vi "Dashboard Main.vi"() -> ()   [LabVIEW 2016]
uses:
  <vilib>/Utility/miscctls.llb/LVRowAndColumnTypeDef.ctl
  <vilib>/event_ctls.llb/eventvkey.ctl
  <vilib>/Rock Robotics/Network Tables/NT Read Boolean.vi
  <vilib>/Rock Robotics/WPI/Dashboard/WPI_DashboardLogging Global.vi
panel:
  in  "Camera Settings Right":T1={"Frame Rate"=30, "Compression"=30, "Size"=1, "DB Camera Config"=FALSE} {"Frame Rate" scale=1.0..30.0; "Compression" scale=100.0..-1.0; "Size" items=["640x480", "320x240", "160x120"]}
  in  "Camera Name Right":string(combo)="No Camera Selection"
  out "Camera Info":cluster{"Mbps LED":bool, "Mbps":dbl, "fps":dbl} {"fps" format="%#.1g"; "Mbps" format="%#.1g"}
  in  "Camera Settings":T1={"Frame Rate"=30, "Compression"=30, "Size"=1, "DB Camera Config"=FALSE} {"Frame Rate" scale=1.0..30.0; "Compression" scale=100.0..-1.0; "Size" items=["640x480", "320x240", "160x120"]}
  in  "TCP":refnum<k5>
  in  "Rec Mode":enum32{"Stop", "Record", "Playback"}(radio)
  out "Robot IP":string
  out "Image Message":string="Timeout in Camera Communications"
  in  "Dashboard Tab":T2(tab)
  in  "Wheel Circumference":dbl=14.0
  in  "?":string(combo)
  out "?":string="CHOOSE AN AUTONOMOUS MODE!!!"
  in  "Select Auto":string(combo)="Select Autonomous ..."
  out "NT Connection":bool
  out "JS1 Z":dbl(slide) scale=-1.0..1.0 scale format="%#_2e"
  out "JS1 Graph":cluster{"X":dbl, "Y":dbl}[](graph)
  out "JS1 Buttons":T3
  out "JS2 Z":dbl(slide) scale=-1.0..1.0 scale format="%#_2e"
  out "JS2 Graph":cluster{"X":dbl, "Y":dbl}[](graph)
  out "JS2 Buttons":T3
  out "Mode":T4(ring)=enum."Auto Disabled"
  out "Camera Image Right":T5(plugin-control)
  out "Gear In?":bool
  in  "?":string="CORTECHS ROBOTICS"
  out "Mid":dbl(slide) scale=0.0..320.0
  out "Targets Found?":bool
  out "Low Gear?":bool
  out "PID On?":bool
  out "?":dbl
  out "Time Remaining":u8(slide) scale=0.0..135.0
  in  "Test Slider":dbl(slide) scale=0.0..100.0 scale format="%#_3g"
  in  "On/Off":bool caption="Solenoid"
  in  "Test Name":u16(ring) items=["Select the test to run..."]
  in  "Test Tree":string(tree)
  in  "Motor":cluster{"Value":dbl, "Enable":bool} {"Value" scale=-1.0..1.0 scale format="%#_3g"}
  out "Progress":T6 {"Test Progress" scale=0.0..100.0}
  in  "Rev/Fwd":cluster{"Forward":bool, "Reverse":bool}
  in  "Test Ring":u16(ring) items=["Monochrome", "Color"]
  out "Cmd Status":string
  in  "Execute Command":bool
  in  "Command Params":string[][](table)
  in  "Command Selection":i32(listbox)
  in  "CheckList":i32(listbox)
  out "Tree":string(tree)
  out "Camera Image":T5(plugin-control)
  out "Background":bool
  in  "Camera Name":string(combo)="No Camera Selection"
  # "HW"
  # "HW"
  # "Joysticks"
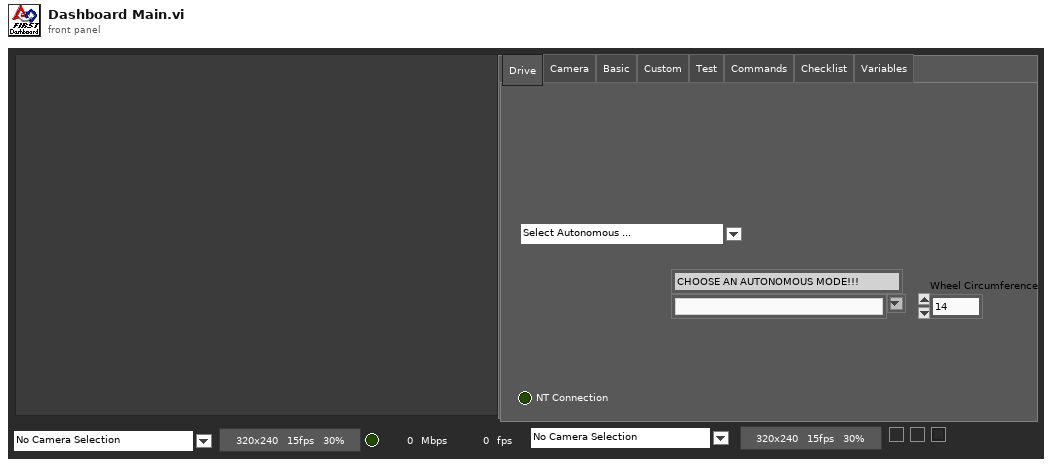
[diagram p1: front panel]
types:
  T1 = cluster{"Frame Rate":i32, "Compression":i32, "Size":u16, "DB Camera Config":bool}
  T2 = enum32{"Drive", "Camera", "Basic", "Custom", "Test", "Commands", "Checklist", "Variables"}
  T3 = cluster{bool, bool, bool, bool, bool, bool, bool, bool, bool, bool, bool, bool}
  T4 = enum8{"Tele-Op Disabled", "Tele-Op Enabled", "Auto Disabled", "Auto Enabled", "Test Disabled", "Test Enabled", "Disconnected", "No Code", "E-Stop"}
  T5 = typedef "IMAQ Image.ctl" = refnum<image>
  T6 = cluster{"Test Progress":u8, "Test Progress Text":string}
  T7 = typedef "Image Type" = u32
  T8 = cluster{"IDs":cluster{"RPC field ID":u16, "Unique ID":u16}, "String":string}
  T9 = enum32{"Drive", "Basic", "Custom", "Test", "Checklist", "Variables"}
  T10 = cluster{"Error Strings":string, "Disable Counts":cluster{u16, u16}, "Rail Faults":cluster{u16, u16, u16}, "Robot IP":string, "DB Mode":u8, "Event Info":cluster{"Name":string, "Type":u8, "Number":u16, "Replay":u8}}
  T11 = cluster{"Storage":cluster{"Disk Free":u64, "RAM Block":u32, "RAM free":u32}, "CPU Utilization":cluster{"CPU % ISR":sgl, "CPU % Time Crit":sgl, "CPU % Timed Str":sgl, "CPU % High":sgl, "CPU % Above":sgl, "CPU % Normal":sgl, "CPU % Low":sgl}, "CAN":cluster{"% Bus Utilization":sgl, "Bus Off Cnt":u32, "TX_FIFO Full Cnt":u32, "Receive Error Cnt":u8, "Transmit Error Cnt":u8}, "HID":cluster{"HID Outputs":u32, "Rumble Low":u16, "Rumble High":u16}[]}
  T12 = cluster{"Status bits":cluster{"Test Mode":bool, "Autonomous":bool, "Enabled":bool, "Code Start":bool, "Brownout":bool, "Reserved 2":bool, "Reserved 3":bool, "E-Stop":bool}, "Code Trace":cluster{"Disabled":bool, "TeleOp":bool, "Auto":bool, "Test":bool}, "Controller Type":enum16{"unknown", "cRIO", "roboRio"}, "Code?":enum16{"unknown", "noCode", "code"}, "Battery V":dbl}
  T13 = cluster{"Control Bits":cluster{"TestMode":bool, "Autonomous":bool, "Enabled":bool, "FMS Present":bool, bool, bool, bool, "E-Stop":bool}, "Team Station ":u8, "Countdown":sgl, "Joystick Values":cluster{"Axes":dbl[], "Buttons":bool[], "POVs":i16[]}[]}
  T14 = cluster{"Axes":dbl[], "Buttons":bool[], "POVs":i16[]}[]
  T15 = cluster{"Axes":dbl[], "Buttons":bool[], "POVs":i16[]}
  T16 = cluster{"Buttons[0]":bool, "Buttons[1]":bool, "Buttons[2]":bool, "Buttons[3]":bool, "Buttons[4]":bool, "Buttons[5]":bool, "Buttons[6]":bool, "Buttons[7]":bool, "Buttons[8]":bool, "Buttons[9]":bool, "Buttons[10]":bool, "Buttons[11]":bool}
  T17 = cluster{"Camera Image":refnum<vi>, "Dashboard Tab":refnum<vi>, "Background":refnum<vi>, "Rec Mode":refnum<vi>, "Test Slider":refnum<vi>, "On/Off ":refnum<vi>, "Test Ring":refnum<vi>, "Rev/Fwd":refnum<vi>, "Test Name":refnum<vi>, "Motor":refnum<vi>, "Progress":refnum<vi>, "CheckList":refnum<vi>, "Tree":refnum<vi>, "Test Tree":refnum<vi>, "Command Params":refnum<vi>, "Command Selection":refnum<vi>, "Execute Command":refnum<vi>, "Cmd Status":refnum<vi>, "Camera Settings":refnum<vi>, "Camera Name":refnum<vi>, "Camera Info":refnum<vi>, "Camera Settings Right":refnum<vi>, "Camera Name Right":refnum<vi>, "Camera Image Right":refnum<vi>}
  T18 = cluster{"Operation":enum16{"Update", "Clear"}, "Color Box":u32}[]
  T19 = typedef "eventvkey.ctl" = enum16{"ASCII", "Enter", "Return", "Shift", "Ctrl", "Alt", "Cmd", "Opt", "Caps", "NumLock", "Clear", "Break", "Up", "Down", "Left", "Right", "Insert", "Delete", "Home", "End", "PageUp", "PageDown", "Escape", "Help", "Pause", "ScrollLock", "F1", "F2", "F3", "F4", "F5", "F6", "F7", "F8", "F9", "F10", "F11", "F12", "F13", "F14", "F15", "F16", "F17", "F18", "F19", "F20", "F21", "F22", "F23", "F24", "Play", "VolumeUp", "VolumeDown", "Mute", "Two Byte Char"}
  T20 = cluster{"Image Size":bool, "Image Type":bool, "Pixel Value":bool, "ROI Information":bool, "Zoom Factor":bool}
  T21 = cluster{"Operation":enum16{"Update", "Clear"}, "Color Box":u32}
  T22 = typedef "LVRowAndColumnTypeDef.ctl" = cluster{"Row":i32, "Column":i32}
  T23 = cluster{"Shift":bool, "Ctrl":bool, "Alt":bool, "Cmd":bool, "Opt":bool}
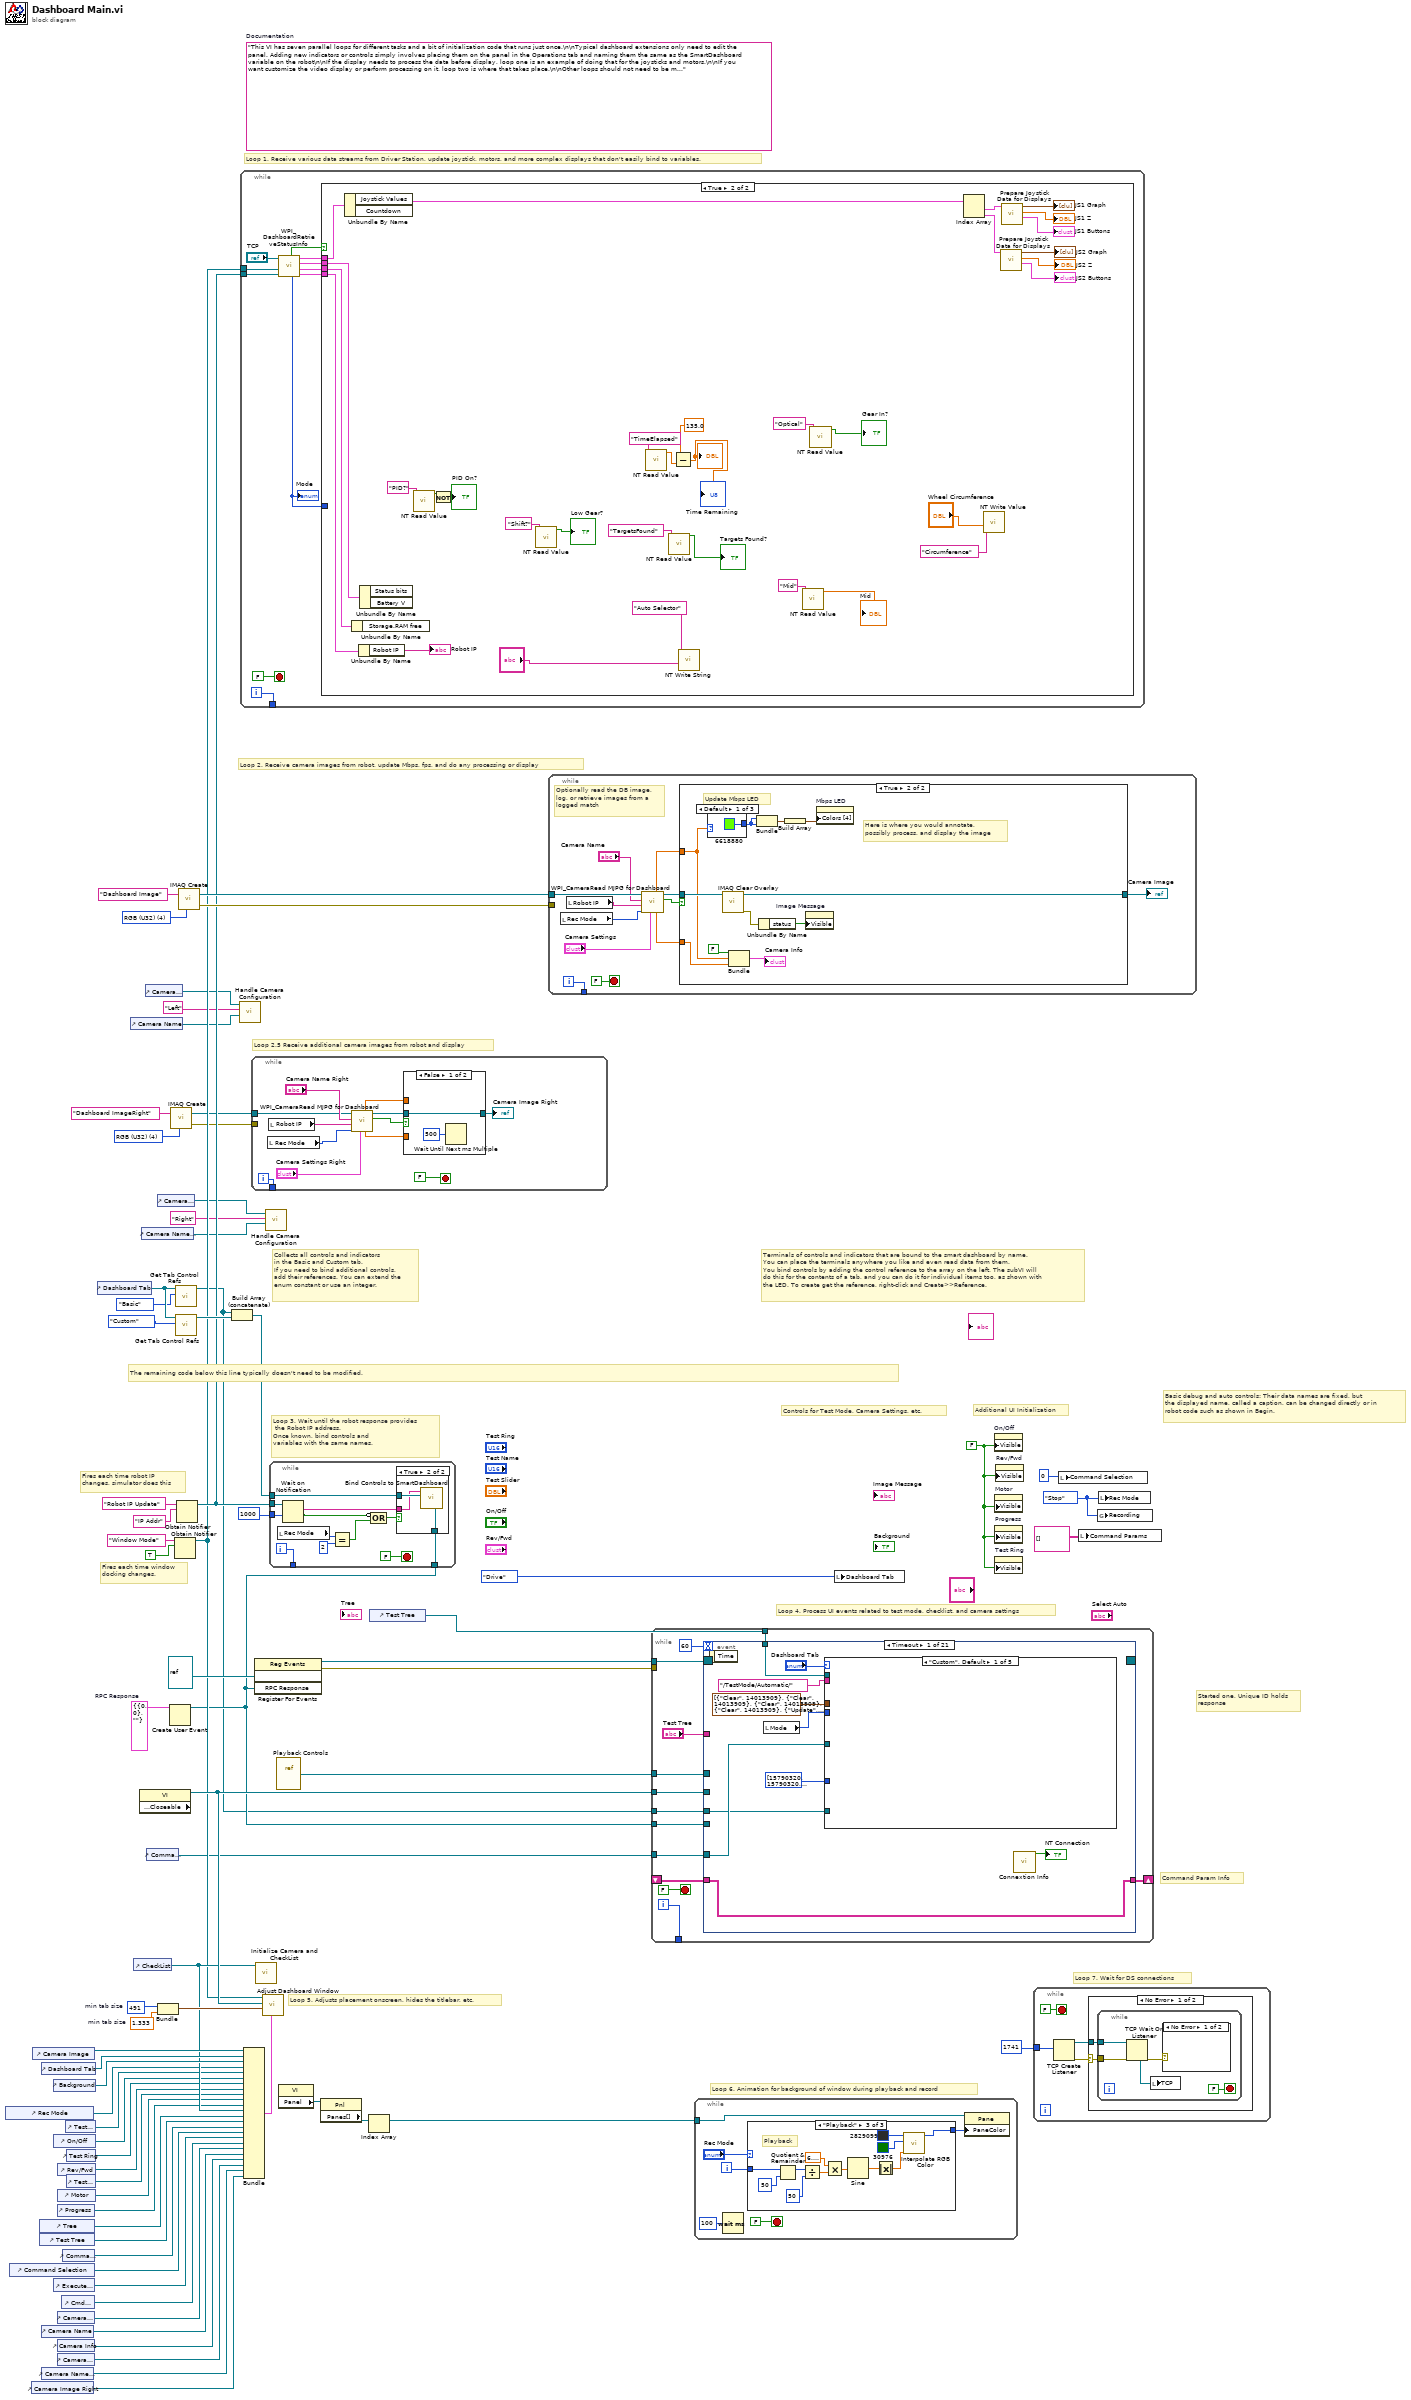
[diagram p0: block diagram]
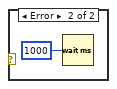
[diagram p3: hidden frame]
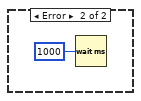
[diagram p4: hidden frame]
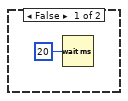
[diagram p5: hidden frame]
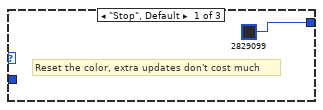
[diagram p6: hidden frame]
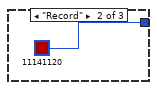
[diagram p7: hidden frame]
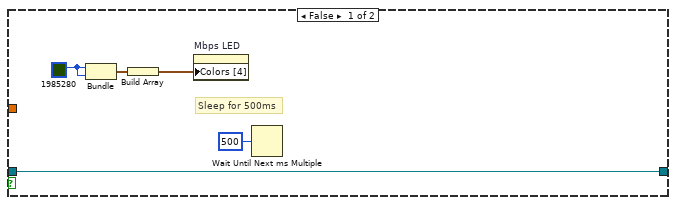
[diagram p9: hidden frame]
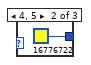
[diagram p10: hidden frame]
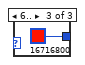
[diagram p11: hidden frame]
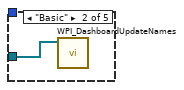
[diagram p12: hidden frame]
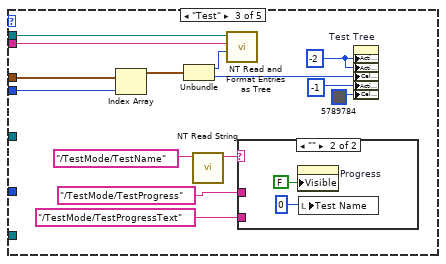
[diagram p13: hidden frame]
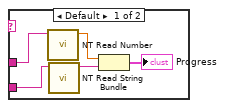
[diagram p14: hidden frame]
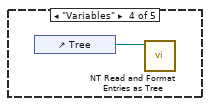
[diagram p15: hidden frame]
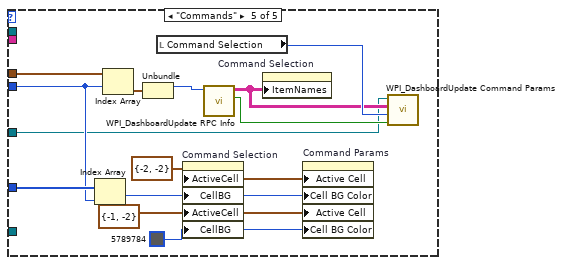
[diagram p16: hidden frame]
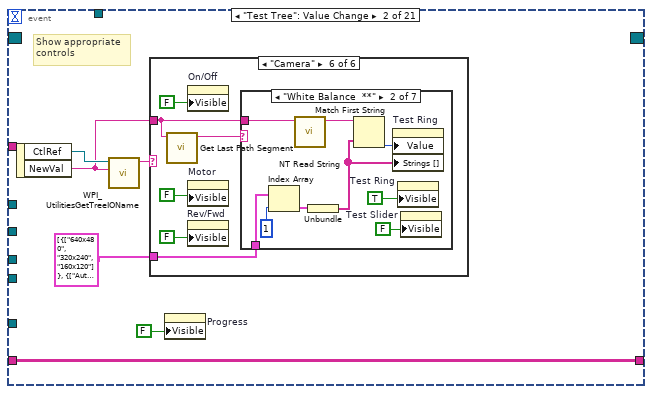
[diagram p17: hidden frame]
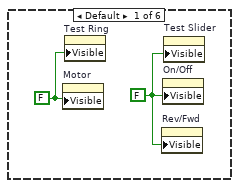
[diagram p18: hidden frame]
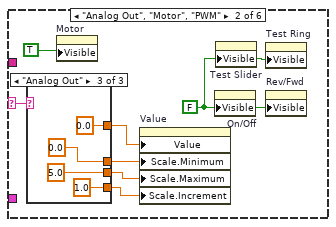
[diagram p19: hidden frame]
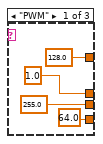
[diagram p20: hidden frame]
diagram:
  w10 = T7 4 items=["Grayscale (U8)", "Grayscale (I16)", "Grayscale (SGL)", "Complex (CSG)", "RGB (U32)", "HSL (U32)", "RGB (U64)"] ("Image Type")
  w24 = T8 {"IDs"={"RPC field ID"=0, "Unique ID"=0}, "String"=""}  # RPC Response
  w49 = 491  # min tab size
  w48 = 1.333  # min tab size
  w56 = enum32{"Stop", "Record", "Playback"}."Stop" ("Rec Mode")
  w31 = FALSE ("Visible")
  (unwired) "This VI has seven parallel loops for different tasks and a bit of initialization code that runs just once.\n\nTypical dashboard extensions only need to edit the panel. Adding new indicators or controls simply involves placing them on the panel in the Operations tab and naming them the same as the SmartDashboard variable on the robot\n\nIf the display needs to process the data before display, loop one is an example of doing that for the joysticks and motors.\n\nIf you want customize the video display or perform processing on it, loop two is where that takes place.\n\nOther loops should not need to be modified. They are pretty standard, and document the task they perform."  # Documentation
  w73 = T7 4 items=["Grayscale (U8)", "Grayscale (I16)", "Grayscale (SGL)", "Complex (CSG)", "RGB (U32)", "HSL (U32)", "RGB (U64)"] ("Image Type")
  # "Loop 2.5 Receive additional camera images from robot and display"
  # "Command Param Info"
  # "Started one, Unique ID holds\nresponse"
  # "Loop 7. Wait for DS connections"
  # "Basic debug and auto controls: Their data names are fixed, but\nthe displayed name, called a caption, can be changed directly or in\nrobot code such as shown in Begin."
  # "Controls for Test Mode, Camera Settings, etc."
  # "Additional UI Initialization"
  # "Loop 6. Animation for background of window during playback and record"
  # "Fires each time robot IP\nchanges, simulator does this"
  # "Fires each time window\ndocking changes."
  # "Collects all controls and indicators\nin the Basic and Custom tab.\nIf you need to bind additional controls,\nadd their references. You can extend the\nenum constant or use an integer."
  # "The remaining code below this line typically doesn't need to be modified."
  # "Loop 4. Process UI events related to test mode, checklist, and camera settings"
  # "Terminals of controls and indicators that are bound to the smart dashboard by name.\nYou can place the terminals anywhere you like and even read data from them.\nYou bind controls by adding the control reference to the array on the left. The subVI will\ndo this for the contents of a tab, and you can do it for individual items too, as shown with\nthe LED. To create get the reference, right-click and Create>>Reference."
  # "Loop 3. Wait until the robot response provides\n the Robot IP address.\nOnce known, bind controls and\nvariables with the same names."
  # "Loop 5. Adjusts placement onscreen, hides the titlebar, etc."
  # "Loop 1. Receive various data streams from Driver Station, update joystick, motors, and more complex displays that don't easily bind to variables."
  # "Loop 2. Receive camera images from robot, update Mbps, fps, and do any processing or display"
  n1 = control-ref of="Rec Mode"() -> (w37:refnum<vi>)
  n2 = control-ref of="Command Selection"() -> (w23:refnum<vi>)
  n3 = control-ref of="Camera Image Right"() -> (w1:refnum<vi>)
  n4 = control-ref of="Camera Image"() -> (w51:refnum<vi>)
  n5 = control-ref of="Tree"() -> (w41:refnum<vi>)
  n6 = control-ref of="Test Tree"() -> (w40:refnum<vi>)
  n7 = control-ref of="Dashboard Tab"() -> (w50:refnum<vi>)
  n8 = control-ref of="Camera Name"() -> (w14:refnum<vi>)
  n9 = control-ref of="Camera Name Right"() -> (w2:refnum<vi>)
  n10 = control-ref of="Execute Command"() -> (w25:refnum<vi>)
  n11 = control-ref of="Background"() -> (w46:refnum<vi>)
  n12 = control-ref of="On/Off"() -> (w35:refnum<vi>)
  n13 = control-ref of="Progress"() -> (w32:refnum<vi>)
  n14 = control-ref of="Camera Settings"() -> (w15:refnum<vi>)
  n15 = control-ref of="Camera Info"() -> (w13:refnum<vi>)
  n16 = control-ref of="Camera Settings Right"() -> (w3:refnum<vi>)
  n17 = control-ref of="Rev/Fwd"() -> (w33:refnum<vi>)
  n18 = control-ref of="Motor"() -> (w38:refnum<vi>)
  n19 = control-ref of="Cmd Status"() -> (w19:refnum<vi>)
  n20 = control-ref of="Command Params"() -> (w26:refnum<vi>)
  n21 = control-ref of="Test Slider"() -> (w36:refnum<vi>)
  n22 = control-ref of="Test Ring"() -> (w34:refnum<vi>)
  n23 = control-ref of="Test Name"() -> (w39:refnum<vi>)
  n24 = control-ref of="Dashboard Tab"() -> (w54:refnum<vi>)
  n25 = control-ref of="Camera Name"() -> (w16:refnum<vi>)
  n26 = control-ref of="CheckList"() -> (w42:refnum<vi>)
  n27 = property class="VI" props=["Front Panel.Closeable"]() -> (reference out=w55:refnum<vi>)  [unwired: 2 in, 2 out]
  n28 = control-ref of="Camera Name Right"() -> (w6:refnum<vi>)
  n29 = control-ref of="Camera Settings"() -> (w17:refnum<vi>)
  n30 = control-ref of="Command Params"() -> (w18:refnum<vi>)
  n31 = control-ref of="Camera Settings Right"() -> (w7:refnum<vi>)
  n32 = Bundle("min tab size"=w49, "min tab size"=w48) -> (w47:cluster{"min tab size":i32, "min tab size":dbl})  [unwired: 1 in]
  n33 = Create User Event(user event datatype=w24) -> (user event=w20:refnum<user-event>)  [unwired: 1 in, 1 out]
  n34 = call "IMAQ Create"("Image Name"="Dashboard ImageRight", "Image Type"=w10) -> ("New Image"=w9:T5, "error out"=w8:errorcluster)  [unwired: 2 in, 1 out]
  n35 = Obtain Notifier(name (unnamed)="Window Mode", notification data type=TRUE) -> (notifier out=w29:refnum<notifier>)  [unwired: 2 in, 2 out]
  n36 = call <vilib>:"Get Tab Control Refs.vi"("Page Index"=T9."Basic" ("Dashboard Tab"), "TabControl in"=w54) -> ("ControlsOnPage"=w12:refnum<vi>[])  [unwired: 9 in]
  n37 = call <vilib>:"Get Tab Control Refs.vi"("Page Index"=T9."Custom" ("Dashboard Tab"), "TabControl in"=w54) -> ("ControlsOnPage"=w53:refnum<vi>[])  [unwired: 9 in]
  n38 = Obtain Notifier(name (unnamed)="Robot IP Update", notification data type="IP Addr" ("name (unnamed)")) -> (notifier out=w30:refnum<notifier>)  [unwired: 2 in, 2 out]
  n39 = call "IMAQ Create"("Image Name"="Dashboard Image", "Image Type"=w73) -> ("New Image"=w71:T5, "error out"=w70:errorcluster)  [unwired: 2 in, 1 out]
  n40 = Build Array (concatenate)(w12, w53) -> (w52:refnum<vi>[])
  n41 = call "Handle Camera Configuration.vi"("CameraNameRef"=w16, "Camera File Name"="Left", "ClusterRef"=w17) -> ()  [unwired: 9 in]
  n42 = while {
    tunnel: [w83] -> _
    tunnel: w30 -> [w77]
    tunnel: w29 -> [w74]
    i -> [w83]
    stop <- FALSE stop-if-true
    n43 = call <vilib>:"WPI_DashboardRetrieveStatusInfo.vi"("Binding Refnum"=w77, "Window Mode Notifier"=w74, "TCP Cnx"="TCP") -> ("Power and Errors"=w78:T10, "Robot Metrics"=w81:T11, "Status Info"=w82:T12, "Control Info"=w79:T13, "Robot Mode"=w76:T4, "Process?"=w80:bool)  [unwired: 3 in]
    "Mode" <- w76
    n44 = case shown="True" w80 {
      tunnel: w82 -> [_ w118]
      tunnel: w81 -> [_ w117]
      tunnel: w79 -> [_ w116]
      tunnel: w78 -> [_ w115]
      tunnel: w76 -> [_ _]
      frame False {
        n45 = Wait (ms)(milliseconds to wait=u32 20) -> ()  [unwired: 1 out]
      }
      frame True {
        n46 = Unbundle By Name(w116) -> ("Joystick Values"=w114:T14)  [unwired: 1 out]
        n47 = Unbundle By Name(w117) -> ()  [unwired: 1 out]
        n48 = Unbundle By Name(w115) -> ("Robot IP"=→"Robot IP":string)
        n49 = Unbundle By Name(w118) -> ()  [unwired: 2 out]
        n50 = call-poly <vilib>:"NT Read Value.vi"("Name"="PID?") -> ("Boolean"=w101:bool)  [unwired: 9 in, 1 out]
        n51 = Not(x=w101) -> (.not. x?=→"PID On?":bool)
        n52 = call-poly <vilib>:"NT Read Value.vi"("Name"="Shift?") -> ("Boolean"=→"Low Gear?":bool)  [unwired: 9 in, 1 out]
        n53 = call-poly <vilib>:"NT Read Value.vi"("Name"="TimeElapsed") -> ("Numeric"=w95:dbl)  [unwired: 9 in, 1 out]
        n54 = call-poly <vilib>:"NT Read Value.vi"("Name"="TargetsFound") -> ("Boolean"=→"Targets Found?":bool)  [unwired: 9 in, 1 out]
        n55 = Subtract(x=135.0, y=w95) -> (x-y=→"Time Remaining" →"?":dbl)
        n56 = call <vilib>:"NT Write String.vi"("String"="?", "Name"="Auto Selector") -> ()  [unwired: 9 in, 1 out]
        n57 = call-poly <vilib>:"NT Read Value.vi"("Name"="Mid") -> ("Numeric"=→"Mid":dbl)  [unwired: 9 in, 1 out]
        n58 = call-poly <vilib>:"NT Read Value.vi"("Name"="Optical") -> ("Boolean"=→"Gear In?":bool)  [unwired: 9 in, 1 out]
        n59 = Index Array(array=w114) -> (element #1=w113:T15, element #2=w109:T15)  [unwired: 2 in]
        n60 = call-poly <vilib>:"NT Write Value.vi"("Numeric"="Wheel Circumference", "Name"="Circumference") -> ()  [unwired: 9 in, 1 out]
        n61 = call "Prepare Joystick Data for Displays.vi"("Joystick Values"=w109) -> ("Buttons"=→"JS2 Buttons":T16, "Z Axis"=→"JS2 Z":dbl, "Cartesian Data"=→"JS2 Graph":cluster{"X axis":dbl, "X axis":dbl}[])  [unwired: 8 in]
        n62 = call "Prepare Joystick Data for Displays.vi"("Joystick Values"=w113) -> ("Buttons"=→"JS1 Buttons":T16, "Z Axis"=→"JS1 Z":dbl, "Cartesian Data"=→"JS1 Graph":cluster{"X axis":dbl, "X axis":dbl}[])  [unwired: 8 in]
      }
    }
  }
  n63 = Bundle("Camera Image"=w51, "Dashboard Tab"=w50, "Background"=w46, "Rec Mode"=w37, "Test Slider"=w36, "On/Off"=w35, "Test Ring"=w34, "Rev/Fwd"=w33, "Test Name"=w39, "Motor"=w38, "Progress"=w32, "CheckList"=w42, "Tree"=w41, "Test Tree"=w40, "Command Params"=w26, "Command Selection"=w23, "Execute Command"=w25, "Cmd Status"=w19, "Camera Settings"=w15, "Camera Name"=w14, "Camera Info"=w13, "Camera Settings Right"=w3, "Camera Name Right"=w2, "Camera Image Right"=w1) -> (w43:T17)  [unwired: 1 in]
  n64 = while {
    tunnel: w9 -> [w129]
    tunnel: w8 -> [_]
    tunnel: [w123] -> _
    i -> [w123]
    stop <- FALSE stop-if-true
    n65 = local read "Rec Mode"() -> (w127:enum32{"Stop", "Record", "Playback"})
    n66 = local read "Robot IP"() -> (w128:string)
    n67 = call <vilib>:"WPI_CameraRead MJPG for Dashboard.vi"("Camera Settings"="Camera Settings Right", "Rec Mode"=w127, "Robot IP"=w128, "Camera Name"="Camera Name Right", "Refnum in"=w129) -> ("Active"=w122:bool, "Refnum out"=w125:T5, "FPS"=w120:dbl, "Bandwidth (Mbps)"=w121:dbl)  [unwired: 3 in]
    n68 = case shown="False" w122 {
      tunnel: w125 -> [w131 w133]
      tunnel: w121 -> [_ _]
      tunnel: w120 -> [_ _]
      tunnel: [w131 w133] -> w119
      frame False {
        n69 = Wait Until Next ms Multiple(millisecond multiple=u32 500) -> ()  [unwired: 1 out]
      }
      frame True {
      }
    }
    "Camera Image Right" <- w119
  }
  n70 = register-events(refnum<vi> refnum, w20) -> (reference out=w60:refnum<event-registration>, error out=w59:errorcluster)  [unwired: 2 in]
  n71 = call "Initialize Camera and CheckList.vi"("ListBox in"=w42) -> ()  [unwired: 11 in]
  n72 = call "Adjust Dashboard Window.vi"("Sizing Refnums"=w43, "Size Constraints"=w47, "VI"=w55, "WIn Mode"=w29) -> ()  [unwired: 8 in]
  n73 = call "Handle Camera Configuration.vi"("CameraNameRef"=w6, "Camera File Name"="Right", "ClusterRef"=w7) -> ()  [unwired: 9 in]
  n74 = while {
    tunnel: w52 -> [w145]
    tunnel: w30 -> [w143]
    tunnel: [w141] -> _
    tunnel: u32 1000 ("milliseconds to wait") -> [w140]
    tunnel: w20 -> [w134]
    i -> [w141]
    stop <- FALSE stop-if-true
    n75 = local read "Rec Mode"() -> (w136:enum32{"Stop", "Record", "Playback"})
    n76 = Wait on Notification(notifier=w143, timeout in ms (-1)=w140) -> (notification=w142:string, timed out?=w138:bool)  [unwired: 2 in, 2 out]
    n77 = Equal?(x=w136, y=u16 2 ("Rec Mode")) -> (x = y?=w137:bool)
    n78 = Compound Arithmetic op=OR(invert w138, w137) -> (w139:bool)
    n79 = case shown="True" w139 {
      tunnel: w145 -> [_ w148]
      tunnel: w142 -> [_ w147]
      tunnel: w134 -> [_ w146]
      frame False {
      }
      frame True {
        n80 = call <vilib>:"Bind Controls to SmartDashboard.vi"("RPC ref"=w146, "Bound Control Refs"=w148, "Server IP Address"=w147) -> ()  [unwired: 9 in]
      }
    }
  }
  n81 = vi-ref "Playback Controls.vi"() -> (w61:refnum<vi>)
  n82 = property class="VI"() -> ("Panel"=w63:refnum<vi>)  [unwired: 2 in, 2 out]
  n83 = property class="Pnl"(reference=w63) -> ("Panes[]"=w64:refnum<vi>[])  [unwired: 1 in, 2 out]
  n84 = Index Array(array=w64) -> (element=w62:refnum<vi>)  [unwired: 1 in]
  n85 = control-ref of="Test Tree"() -> (w65:refnum<vi>)
  n86 = while {
    tunnel: w71 -> [w158]
    tunnel: w70 -> [_]
    tunnel: [w159] -> _
    i -> [w159]
    stop <- FALSE stop-if-true
    # "Optionally read the DB image,\nlog, or retrieve images from a\nlogged match"
    n87 = local read "Rec Mode"() -> (w154:enum32{"Stop", "Record", "Playback"})
    n88 = local read "Robot IP"() -> (w153:string)
    n89 = call <vilib>:"WPI_CameraRead MJPG for Dashboard.vi"("Camera Settings"="Camera Settings", "Rec Mode"=w154, "Robot IP"=w153, "Camera Name"="Camera Name", "Refnum in"=w158) -> ("Active"=w156:bool, "Refnum out"=w157:T5, "FPS"=w155:dbl, "Bandwidth (Mbps)"=w152:dbl)  [unwired: 3 in]
    n90 = case shown="True" w156 {
      tunnel: w157 -> [w161 w172]
      tunnel: w152 -> [_ w169]
      tunnel: w155 -> [_ w170]
      tunnel: [w161 w166] -> w149
      frame False {
        w163 = u32 1985280 ("Color Box")
        # "Sleep for 500ms"
        n91 = Bundle("Color Box"=w163, "Color Box"=w163) -> (w164:cluster{"Color Box":u32, "Color Box":u32})  [unwired: 1 out]
        n92 = Build Array(w164) -> (w162:cluster{"Color Box":u32, "Color Box":u32}[])
        n93 = property on="Mbps LED" class="Bool (strict)"("Colors [4]"=w162) -> ()  [unwired: 2 in, 2 out]
        n94 = Wait Until Next ms Multiple(millisecond multiple=u32 500) -> ()  [unwired: 1 out]
      }
      frame True {
        # "Here is where you would annotate,\npossibly process, and display the image"
        # "Update Mbps LED"
        n95 = case shown="Default" w169 {
          tunnel: [u32 6618880 ("Color Box") u32 16776722 ("Color Box") u32 16716800 ("Color Box")] -> w173
          frame Default {
          }
          frame 4, 5 {
          }
          frame 6.. {
          }
        }
        n96 = call "IMAQ Clear Overlay"("Image"=w172) -> ("error out"=w175:errorcluster, "Image Out"=w166:T5)  [unwired: 2 in, 7 out]
        n97 = Bundle(FALSE, "Bandwidth (Mbps)"=w169, "FPS"=w170) -> (→"Camera Info":cluster{bool, "Bandwidth (Mbps)":dbl, "FPS":dbl})  [unwired: 1 in]
        n98 = Bundle("Color Box"=w173, "Color Box"=w173) -> (w174:cluster{"Color Box":u32, "Color Box":u32})  [unwired: 1 out]
        n99 = Unbundle By Name(w175) -> ("status"=w176:bool)
        n100 = Build Array(w174) -> (w171:cluster{"Color Box":u32, "Color Box":u32}[])
        n101 = property on="Image Message" class="Str"("Visible"=w176) -> ()  [unwired: 2 in, 2 out]
        n102 = property on="Mbps LED" class="Bool (strict)"("Colors [4]"=w171) -> ()  [unwired: 2 in, 2 out]
      }
    }
    "Camera Image" <- w149
  }
  n103 = while {
    tunnel: [w189] -> _
    tunnel: w65 -> [w188]
    tunnel: w61 -> [w187]
    tunnel: w60 -> [w186]
    tunnel: w59 -> [_]
    tunnel: w55 -> [w185]
    tunnel: w20 -> [w184]
    tunnel: w18 -> [w183]
    shift-right: [w182] -> _
    shift-left: _ -> [w181]
    tunnel: w12 -> [w180]
    i -> [w189]
    stop <- FALSE stop-if-true
    n104 = event shown="[0] Timeout" {
      selector: w186 -> [_ _ _ _ _ _ _ _ _ _ _ _ _ _ _ _ _ _ _ _ _]
      dyn-events: [_ _ _ _ _ _ _ _ _ _ _ _ _ _ _ _ w445 _ _ _ _] -> _
      timeout: u32 60 ("milliseconds to wait") -> [_ _ _ _ _ _ _ _ _ _ _ _ _ _ _ _ _ _ _ _ _]
      tunnel: w188 -> [w201 _ _ _ _ _ _ _ _ _ _ _ _ _ _ _ _ _ _ _ _]
      tunnel: "Test Tree" -> [_ _ _ _ _ _ _ _ _ _ _ w412 w420 w422 w426 w434 _ _ _ _ _]
      tunnel: w187 -> [_ _ _ _ _ _ _ _ _ _ _ _ _ _ _ _ w447 _ w465 _ _]
      tunnel: w185 -> [_ _ _ _ _ _ _ _ _ _ _ _ _ _ _ _ w443 _ _ _ _]
      tunnel: w184 -> [_ _ _ _ _ _ _ _ _ _ _ _ _ _ _ _ w439 _ _ _ _]
      tunnel: w183 -> [w196 _ _ _ _ _ w363 _ _ _ _ _ _ _ _ _ _ _ _ _ _]
      tunnel: [w195 w240 w342 w347 w356 w360 w361 w370 w380 w387 w399 w411 w418 w421 w425 w433 w438 w460 w462 w466 w477] -> w182
      tunnel: w181 -> [w195 w240 w342 w347 w356 w360 w361 _ _ w387 w399 w411 w418 w421 w425 w433 w438 w460 w462 w466 w477]
      tunnel: w180 -> [w193 _ _ _ _ _ _ _ _ _ _ _ _ _ _ _ _ _ _ _ _]
      event Timeout {
        n105 = event-data() -> ()  [unwired: 1 in, 1 out]
        n106 = local read "Mode"() -> (w198:T4)
        n107 = case shown="\"Custom\", Default" "Dashboard Tab" {
          tunnel: w201 -> [_ _ w217 _ _]
          tunnel: "/TestMode/Automatic/" ("Name Pattern") -> [_ _ w216 _ _]
          tunnel: T18 [{"Operation"=enum."Clear", "Color Box"=14013909}, {"Operation"=enum."Clear", "Color Box"=14013909}, {"Operation"=enum."Clear", "Color Box"=14013909}, {"Operation"=enum."Clear", "Color Box"=14013909}, {"Operation"=enum."Update", "Color Box"=14013909}, {"Operation"=enum."Update", "Color Box"=16777215}, {"Operation"=enum."Clear", "Color Box"=14013909}, {"Operation"=enum."Clear", "Color Box"=14013909}, {"Operation"=enum."Clear", "Color Box"=14013909}] -> [_ _ w209 _ w233]
          tunnel: w198 -> [_ _ w208 _ w232]
          tunnel: u32[] [15790320, 15790320, 15790320, 15790320, 16777215, 16777215, 15790320, 15790320, 15790320] -> [_ _ _ _ w238]
          tunnel: w196 -> [_ _ _ _ w226]
          tunnel: w193 -> [_ w203 _ _ _]
          frame "Custom", Default {
          }
          frame "Basic" {
            n108 = call <vilib>:"WPI_DashboardUpdateNames.vi"("Controls on Tab"=w203) -> ()  [unwired: 11 in]
          }
          frame "Test" {
            w215 = -2 ("Active Item:Row Number")
            n109 = Index Array(array=w209, index=w208) -> (element=w210:T21)
            n110 = Unbundle(w210) -> ("Operation"=w211:enum16{"Update", "Clear"}, "Color Box"=w212:u32)
            n111 = call <vilib>:"NT Read String.vi"("Name"="/TestMode/TestName") -> ("String"=w206:string)  [unwired: 9 in, 1 out]
            n112 = call <vilib>:"NT Read and Format Entries as Tree.vi"("Operation"=w211, "Name Pattern"=w216, "Tree Refnum"=w217) -> ()  [unwired: 7 in, 2 out]
            n113 = case shown="\"\"" w206 {
              tunnel: "/TestMode/TestProgress" ("Name") -> [w219 _]
              tunnel: "/TestMode/TestProgressText" ("Name") -> [w218 _]
              frame Default {
                n114 = call <vilib>:"NT Read Number.vi"("Name"=w219) -> ("Numeric"=w220:dbl)  [unwired: 9 in, 1 out]
                n115 = call <vilib>:"NT Read String.vi"("Name"=w218) -> ("String"=w221:string)  [unwired: 9 in, 1 out]
                n116 = Bundle("Numeric"=w220, "String"=w221) -> (→"Progress":cluster{"Numeric":dbl, "String":string})  [unwired: 1 in]
              }
              frame "" {
                n117 = property on="Progress" class="Clust (strict)"("Visible"=FALSE) -> ()  [unwired: 2 in, 2 out]
                n118 = local write "Test Name"(u16 0) -> ()
              }
            }
            n119 = property on="Test Tree" class="Tree (strict)"("Active Item Row Number"=w215, "ActiveColNum"=w215, "CellBG"=w212, "Active Item Row Number"=-1 ("Active Item:Row Number"), "CellBG"=u32 5789784 ("Color Box")) -> ()  [unwired: 2 in, 2 out]
          }
          frame "Variables" {
            n120 = control-ref of="Tree"() -> (w225:refnum<vi>)
            n121 = call <vilib>:"NT Read and Format Entries as Tree.vi"("Tree Refnum"=w225) -> ()  [unwired: 9 in, 2 out]
          }
          frame "Commands" {
            w234 = u32 5789784 ("Color Box")
            w235 = T22 {"Row"=-1, "Column"=-2} ("Active Cell:Active Cell")
            w237 = T22 {"Row"=-2, "Column"=-2} ("Active Cell:Active Cell")
            n122 = Index Array(array=w238, index=w232) -> (element=w236:u32)
            n123 = Index Array(array=w233, index=w232) -> (element=w231:T21)
            n124 = Unbundle(w231) -> ("Operation"=w230:enum16{"Update", "Clear"})  [unwired: 1 out]
            n125 = local read "Command Selection"() -> (w229:i32)
            n126 = property on="Command Selection" class="MCListbox (strict)"("ActiveCell"=w237, "CellBG"=w236, "ActiveCell"=w235, "CellBG"=w234) -> ()  [unwired: 2 in, 2 out]
            n127 = call <vilib>:"WPI_DashboardUpdate RPC Info.vi"("Operation"=w230) -> ("update"=w228:bool, "commands"=w227:string[][])  [unwired: 9 in]
            n128 = property on="Command Selection" class="MCListbox (strict)"("ItemNames"=w227) -> ()  [unwired: 2 in, 2 out]
            n129 = property on="Command Params" class="Tbl (strict)"("Active Cell"=w237, "Cell BG Color"=w236, "Active Cell"=w235, "Cell BG Color"=w234) -> ()  [unwired: 2 in, 2 out]
            n130 = call <vilib>:"WPI_DashboardUpdate Command Params.vi"("Update"=w228, "NewVal"=w229, "Commands"=w227, "Param Tbl"=w226) -> ()  [unwired: 7 in, 1 out]
          }
        }
        n131 = call <vilib>:"Connextion Info.vi"() -> ("Connected"=→"NT Connection":bool)  [unwired: 10 in, 1 out]
      }
      event "Test Tree": Value Change {
        # "Show appropriate\ncontrols"
        n132 = event-data() -> ("CtlRef"=w243:refnum<vi>, "NewVal"=w241:string)  [unwired: 1 in]
        n133 = call <vilib>:"WPI_UtilitiesGetTreeIOName.vi"("NewVal"=w241, "TreeControl in"=w243) -> ("I/O Name"=w244:string)  [unwired: 9 in]
        n134 = case shown="\"Camera\"" w244 {
          selector: w244 -> [_ w251 _ w273 w282 _]
          tunnel: w241 -> [_ _ w270 w272 _ w289]
          tunnel: cluster{string[]}[] [{["640x480", "320x240", "160x120"]}, {["Auto", "Fixed indoor", "Fixed outdoor 1", "Fixed outdoor 2", "Fixed fluorescent 1", "Fixed fluorescent 2", "Hold current"]}, {["Auto", "Flicker-free 50 Hz", "Flicker-free 60 Hz", "Hold current"]}, {["None", "Prioritize frame rate", "Prioritize image quality"]}, {["Monochrome", "Color"]}] -> [_ _ _ _ _ w288]
          frame Default {
            w246 = FALSE ("Visible")
            w245 = FALSE ("Visible")
            n135 = property on="Motor" class="Clust (strict)"("Visible"=w245) -> ()  [unwired: 2 in, 2 out]
            n136 = property on="Test Ring" class="Ring (strict)"("Visible"=w245) -> ()  [unwired: 2 in, 2 out]
            n137 = property on="Rev/Fwd" class="Clust (strict)"("Visible"=w246) -> ()  [unwired: 2 in, 2 out]
            n138 = property on="On/Off" class="Bool (strict)"("Visible"=w246) -> ()  [unwired: 2 in, 2 out]
            n139 = property on="Test Slider" class="Slide (strict)"("Visible"=w246) -> ()  [unwired: 2 in, 2 out]
          }
          frame "Analog Out", "Motor", "PWM" {
            w252 = FALSE ("Visible")
            n140 = case shown="\"Analog Out\"" w251 {
              tunnel: [1.0 ("Value") -1.0 ("Value") 0.0 ("Value")] -> w250
              tunnel: [255.0 ("Value") 1.0 ("Value") 5.0 ("Value")] -> w249
              tunnel: [128.0 ("Value") 0.0 ("Value") 0.0 ("Value")] -> w248
              tunnel: [64.0 ("Value") 0.5 ("Value") 1.0 ("Value")] -> w247
              frame "PWM" {
              }
              frame "Motor", Default {
              }
              frame "Analog Out" {
              }
            }
            n141 = property on="Motor" class="Clust (strict)"("Visible"=TRUE) -> ()  [unwired: 2 in, 2 out]
            n142 = property on="Value" class="Slide (strict)"("Value"=w248, "Scale.Minimum"=w250, "Scale.Maximum"=w249, "Scale.Increment"=w247) -> ()  [unwired: 2 in, 2 out]
            n143 = property on="On/Off" class="Bool (strict)"("Visible"=w252) -> ()  [unwired: 2 in, 2 out]
            n144 = property on="Test Slider" class="Slide (strict)"("Visible"=w252) -> ()  [unwired: 2 in, 2 out]
            n145 = property on="Test Ring" class="Ring (strict)"("Visible"=w252) -> ()  [unwired: 2 in, 2 out]
            n146 = property on="Rev/Fwd" class="Clust (strict)"("Visible"=w252) -> ()  [unwired: 2 in, 2 out]
          }
          frame "Servo" {
            w268 = FALSE ("Visible")
            n147 = call <vilib>:"NT Read Number.vi"("Name"=w270) -> ("Numeric"=w269:dbl)  [unwired: 9 in, 1 out]
            n148 = property on="Test Slider" class="Slide (strict)"("Visible"=TRUE, "Scale.Maximum"=170.0 ("Scale.Range:Maximum")) -> ()  [unwired: 2 in, 2 out]
            n149 = local write "Test Slider"(w269) -> ()
            n150 = property on="Motor" class="Clust (strict)"("Visible"=w268) -> ()  [unwired: 2 in, 2 out]
            n151 = property on="Rev/Fwd" class="Clust (strict)"("Visible"=w268) -> ()  [unwired: 2 in, 2 out]
            n152 = property on="On/Off" class="Bool (strict)"("Visible"=w268) -> ()  [unwired: 2 in, 2 out]
            n153 = property on="Test Ring" class="Ring (strict)"("Visible"=w268) -> ()  [unwired: 2 in, 2 out]
          }
          frame "Relay", "Solenoid" {
            w271 = FALSE ("Visible")
            n154 = property on="Motor" class="Clust (strict)"("Visible"=w271) -> ()  [unwired: 2 in, 2 out]
            n155 = property on="Test Slider" class="Slide (strict)"("Visible"=w271) -> ()  [unwired: 2 in, 2 out]
            n156 = Search and Replace String(input string=w272, search string="/Value  **", replace string="/Direction") -> (result string=w278:string)  [unwired: 5 in, 3 out]
            n157 = property on="Test Ring" class="Ring (strict)"("Visible"=w271) -> ()  [unwired: 2 in, 2 out]
            n158 = call <vilib>:"NT Read String.vi"("Name"=w278) -> ("String"=w276:string)  [unwired: 9 in, 1 out]
            n159 = Equal?(x="Both directions", y=w276) -> (x = y?=w274:bool)
            n160 = Not(x=w274) -> (.not. x?=w275:bool)
            n161 = property on="Rev/Fwd" class="Clust (strict)"("Visible"=w274) -> ()  [unwired: 2 in, 2 out]
            n162 = property on="On/Off" class="Bool (strict)"("Visible"=w275, "Caption.Text"=w273) -> ()  [unwired: 2 in, 2 out]
          }
          frame "Compressor", "Digital Out" {
            w281 = FALSE ("Visible")
            # "Get direction and finish"
            n163 = property on="Motor" class="Clust (strict)"("Visible"=w281) -> ()  [unwired: 2 in, 2 out]
            n164 = property on="Test Slider" class="Slide (strict)"("Visible"=w281) -> ()  [unwired: 2 in, 2 out]
            n165 = property on="Test Ring" class="Ring (strict)"("Visible"=w281) -> ()  [unwired: 2 in, 2 out]
            n166 = property on="On/Off" class="Bool (strict)"("Visible"=TRUE, "Caption.Text"=w282) -> ()  [unwired: 2 in, 2 out]
            n167 = property on="Rev/Fwd" class="Clust (strict)"("Visible"=FALSE) -> ()  [unwired: 2 in, 2 out]
          }
          frame "Camera" {
            n168 = call <vilib>:"Get Last Path Segment.vi"("String in"=w289) -> ("String out"=w290:string)  [unwired: 10 in]
            n169 = property on="On/Off" class="Bool (strict)"("Visible"=FALSE) -> ()  [unwired: 2 in, 2 out]
            n170 = property on="Motor" class="Clust (strict)"("Visible"=FALSE) -> ()  [unwired: 2 in, 2 out]
            n171 = property on="Rev/Fwd" class="Clust (strict)"("Visible"=FALSE) -> ()  [unwired: 2 in, 2 out]
            n172 = case shown="\"White Balance  **\"" w290 {
              tunnel: w289 -> [w296 w305 w314 w323 w332 _ w338]
              tunnel: w288 -> [w294 w302 w311 w320 w329 _ _]
              frame "Size  **" {
                n173 = Index Array(array=w294) -> (element=w293:cluster{string[]})  [unwired: 1 in]
                n174 = call <vilib>:"NT Read String.vi"("Name"=w296) -> ("String"=w295:string)  [unwired: 9 in, 1 out]
                n175 = Unbundle(w293) -> (w291:string[])
                n176 = Match First String(2:w291, 3:w295) -> (0:w292:i32)  [unwired: 1 out]
                n177 = property on="Test Ring" class="Ring (strict)"("Value"=w292, "Strings []"=w291) -> ()  [unwired: 2 in, 2 out]
                n178 = property on="Test Ring" class="Ring (strict)"("Visible"=TRUE) -> ()  [unwired: 2 in, 2 out]
                n179 = property on="Test Slider" class="Slide (strict)"("Visible"=FALSE) -> ()  [unwired: 2 in, 2 out]
              }
              frame "White Balance  **" {
                n180 = Index Array(array=w302, index=1) -> (element=w303:cluster{string[]})
                n181 = call <vilib>:"NT Read String.vi"("Name"=w305) -> ("String"=w304:string)  [unwired: 9 in, 1 out]
                n182 = Unbundle(w303) -> (w300:string[])
                n183 = Match First String(2:w300, 3:w304) -> (0:w299:i32)  [unwired: 1 out]
                n184 = property on="Test Ring" class="Ring (strict)"("Value"=w299, "Strings []"=w300) -> ()  [unwired: 2 in, 2 out]
                n185 = property on="Test Ring" class="Ring (strict)"("Visible"=TRUE) -> ()  [unwired: 2 in, 2 out]
                n186 = property on="Test Slider" class="Slide (strict)"("Visible"=FALSE) -> ()  [unwired: 2 in, 2 out]
              }
              frame "Exposure  **" {
                n187 = Index Array(array=w311, index=2) -> (element=w312:cluster{string[]})
                n188 = call <vilib>:"NT Read String.vi"("Name"=w314) -> ("String"=w313:string)  [unwired: 9 in, 1 out]
                n189 = Unbundle(w312) -> (w308:string[])
                n190 = Match First String(2:w308, 3:w313) -> (0:w309:i32)  [unwired: 1 out]
                n191 = property on="Test Ring" class="Ring (strict)"("Value"=w309, "Strings []"=w308) -> ()  [unwired: 2 in, 2 out]
                n192 = property on="Test Ring" class="Ring (strict)"("Visible"=TRUE) -> ()  [unwired: 2 in, 2 out]
                n193 = property on="Test Slider" class="Slide (strict)"("Visible"=FALSE) -> ()  [unwired: 2 in, 2 out]
              }
              frame "Exposure Priority  **" {
                n194 = Index Array(array=w320, index=3) -> (element=w321:cluster{string[]})
                n195 = call <vilib>:"NT Read String.vi"("Name"=w323) -> ("String"=w322:string)  [unwired: 9 in, 1 out]
                n196 = Unbundle(w321) -> (w317:string[])
                n197 = Match First String(2:w317, 3:w322) -> (0:w318:i32)  [unwired: 1 out]
                n198 = property on="Test Ring" class="Ring (strict)"("Value"=w318, "Strings []"=w317) -> ()  [unwired: 2 in, 2 out]
                n199 = property on="Test Ring" class="Ring (strict)"("Visible"=TRUE) -> ()  [unwired: 2 in, 2 out]
                n200 = property on="Test Slider" class="Slide (strict)"("Visible"=FALSE) -> ()  [unwired: 2 in, 2 out]
              }
              frame "Color Enable  **" {
                n201 = Index Array(array=w329, index=4) -> (element=w330:cluster{string[]})
                n202 = call <vilib>:"NT Read String.vi"("Name"=w332) -> ("String"=w331:string)  [unwired: 9 in, 1 out]
                n203 = Unbundle(w330) -> (w326:string[])
                n204 = Match First String(2:w326, 3:w331) -> (0:w327:i32)  [unwired: 1 out]
                n205 = property on="Test Ring" class="Ring (strict)"("Value"=w327, "Strings []"=w326) -> ()  [unwired: 2 in, 2 out]
                n206 = property on="Test Ring" class="Ring (strict)"("Visible"=TRUE) -> ()  [unwired: 2 in, 2 out]
                n207 = property on="Test Slider" class="Slide (strict)"("Visible"=FALSE) -> ()  [unwired: 2 in, 2 out]
              }
              frame Default {
                n208 = property on="Test Ring" class="Ring (strict)"("Visible"=FALSE) -> ()  [unwired: 2 in, 2 out]
                n209 = property on="Test Slider" class="Slide (strict)"("Visible"=FALSE) -> ()  [unwired: 2 in, 2 out]
              }
              frame "Brightness  **", "Color Level  **", "Compression  **", "FPS  **", "Sharpness  **" {
                n210 = call <vilib>:"NT Read Number.vi"("Name"=w338) -> ("Numeric"=w337:dbl)  [unwired: 9 in, 1 out]
                n211 = local write "Test Slider"(w337) -> ()
                n212 = property on="Test Slider" class="Slide (strict)"("Visible"=TRUE, "Scale.Maximum"=100.0 ("Scale.Range:Maximum")) -> ()  [unwired: 2 in, 2 out]
                n213 = property on="Test Ring" class="Ring (strict)"("Visible"=FALSE) -> ()  [unwired: 2 in, 2 out]
              }
            }
          }
        }
        n214 = property on="Progress" class="Clust (strict)"("Visible"=FALSE) -> ()  [unwired: 2 in, 2 out]
      }
      event "Test Name": Mouse Enter {
        # "Populate the ring with the list of tests"
        n215 = event-data() -> ()  [unwired: 1 in, 1 out]
        n216 = call <vilib>:"NT Read String Array.vi"("Name"="/TestMode/TestList") -> ("String Array"=w346:string[])  [unwired: 9 in, 1 out]
        n217 = Build Array (concatenate)("Select the test to run...", w346) -> (w345:string[])
        n218 = property on="Test Name" class="Ring (strict)"("Strings []"=w345) -> ()  [unwired: 2 in, 2 out]
      }
      event "Test Name": Value Change {
        w348 = FALSE ("Visible")
        # "Tell the robot the test name to run"
        n219 = event-data() -> ("NewVal"=w352:u16)  [unwired: 1 in]
        n220 = property on="Test Name" class="Ring (strict)"() -> ("Strings []"=w353:string[])  [unwired: 2 in, 2 out]
        n221 = local write "Progress"(T6 {"Test Progress"=0, "Test Progress Text"=""} ("Progress")) -> ()
        n222 = Index Array(array=w353, index=w352) -> (element=w351:string)
        n223 = call <vilib>:"NT Write String.vi"("String"=w351, "Name"="/TestMode/TestName") -> ()  [unwired: 9 in, 1 out]
        n224 = property on="Progress" class="Clust (strict)"("Visible"=TRUE) -> ()  [unwired: 2 in, 2 out]
        n225 = property on="Motor" class="Clust (strict)"("Visible"=w348) -> ()  [unwired: 2 in, 2 out]
        n226 = property on="Test Slider" class="Slide (strict)"("Visible"=w348) -> ()  [unwired: 2 in, 2 out]
        n227 = property on="On/Off" class="Bool (strict)"("Visible"=w348) -> ()  [unwired: 2 in, 2 out]
        n228 = property on="Rev/Fwd" class="Clust (strict)"("Visible"=w348) -> ()  [unwired: 2 in, 2 out]
        n229 = property on="Test Ring" class="Ring (strict)"("Visible"=w348) -> ()  [unwired: 2 in, 2 out]
      }
      event "Select Auto": Mouse Enter {
        # "Populate the combo box with the list of autonomous options"
        n230 = event-data() -> ()  [unwired: 1 in, 1 out]
        n231 = call <vilib>:"NT Read String Array.vi"("Name"="Auto List") -> ("String Array"=w355:string[])  [unwired: 9 in, 1 out]
        n232 = property on="Select Auto" class="CmbBox"("Strings[]"=w355) -> ()  [unwired: 2 in, 2 out]
      }
      event "Select Auto": Value Change {
        # "User modified the Auto Selection. Write to NT variable so robot knows."
        n233 = event-data() -> ("NewVal"=w358:string)  [unwired: 1 in]
        n234 = call <vilib>:"NT Write String.vi"("String"=w358, "Name"="Auto Selector") -> ()  [unwired: 9 in, 1 out]
      }
      event "Command Selection": Value Change {
        # "Get the params and show in table"
        n235 = event-data() -> ("NewVal"=w364:i32)  [unwired: 1 in]
        n236 = property on="Command Selection" class="MCListbox (strict)"() -> ("ItemNames"=w362:string[][])  [unwired: 2 in, 2 out]
        n237 = call <vilib>:"WPI_DashboardUpdate Command Params.vi"("NewVal"=w364, "Commands"=w362, "Param Tbl"=w363) -> ()  [unwired: 8 in, 1 out]
      }
      event "Execute Command": Value Change {
        # "Started one, Unique ID holds\nresponse"
        n238 = event-data() -> ()  [unwired: 1 in, 1 out]
        n239 = property on="Command Selection" class="MCListbox (strict)"() -> ("ItemNames"=w375:string[][])  [unwired: 2 in, 2 out]
        n240 = Index Array(array=w375, index (row)="Command Selection", index (col)=0) -> (element=w373:string)
        n241 = call <vilib>:"Invoke Commands.vi"("Command Params"="Command Params", "Function Name"=w373) -> ("Params"=w369:u8, "Started"=w368:bool)  [unwired: 7 in, 1 out]
        n242 = Array Subset(array="Command Params", length (row)=w369) -> (w370:string[][])  [unwired: 3 in]
        n243 = Select(t="Executing" ("Cmd Status"), s=w368, f="" ("Cmd Status")) -> (s? t:f=→"Cmd Status":string)
      }
      event "Command Selection": Double Click {
        n244 = event-data() -> ("Row"=w383:i32)  [unwired: 1 in]
        n245 = property on="Command Selection" class="MCListbox (strict)"() -> ("ItemNames"=w386:string[][])  [unwired: 2 in, 2 out]
        n246 = local read "Command Params"() -> (w382:string[][])
        n247 = Index Array(array=w386, index (row)=w383, index (col)=0) -> (element=w384:string)
        n248 = call <vilib>:"Invoke Commands.vi"("Command Params"=w382, "Function Name"=w384) -> ("Params"=w381:u8, "Started"=w376:bool)  [unwired: 7 in, 1 out]
        n249 = Array Subset(array=w382, length (row)=w381) -> (w380:string[][])  [unwired: 3 in]
        n250 = Select(t="Executing" ("Cmd Status"), s=w376, f="" ("Cmd Status")) -> (s? t:f=w377:string)
        n251 = local write "Cmd Status"(w377) -> ()
      }
      event "CheckList": Double Click {
        # "Shift clears all"
        # "Update symbols on the listbox"
        n252 = event-data() -> ("PlatMods.Shift"=w388:bool, "Row"=w390:i32)  [unwired: 1 in]
        n253 = case shown="True" w388 {
          tunnel: w390 -> [w394 _]
          tunnel: 1 -> [w393 _]
          frame False {
            n254 = property on="CheckList" class="LstBox (strict)"() -> ("Item Symbols"=w392:i32[])  [unwired: 2 in, 2 out]
            n255 = Replace Array Subset(array=w392, new element=w393, index=w394) -> (w391:i32[])
            n256 = property on="CheckList" class="LstBox (strict)"("Item Symbols"=w391) -> ()  [unwired: 2 in, 2 out]
          }
          frame True {
            w395 = 0 ("Top Row")
            n257 = property on="CheckList" class="LstBox (strict)"() -> ("Number of Rows"=w397:u32)  [unwired: 2 in, 2 out]
            n258 = Initialize Array(0, w397) -> (w396:i32[])
            n259 = property on="CheckList" class="LstBox (strict)"("Top Row"=w395, "Value"=w395, "Item Symbols"=w396) -> ()  [unwired: 2 in, 2 out]
          }
        }
      }
      event "CheckList": Key Down {
        # "Update symbols on the listbox\nLeft and right keys check and uncheck"
        n260 = event-data() -> ("VKey"=w401:T19)  [unwired: 1 in]
        n261 = case shown="\"Left\", \"Right\"" w401 {
          selector: w401 -> [w406 _]
          tunnel: eventvkey."Left" ("VKey") -> [w404 _]
          frame "Left", "Right" {
            n262 = Equal?(x=w404, y=w406) -> (x = y?=w405:bool)
            n263 = Select(t=0, s=w405, f=1) -> (s? t:f=w407:i32)
            n264 = property on="CheckList" class="LstBox (strict)"() -> ("Item Symbols"=w410:i32[])  [unwired: 2 in, 2 out]
            n265 = Replace Array Subset(array=w410, new element=w407, index="CheckList") -> (w409:i32[])
            n266 = property on="CheckList" class="LstBox (strict)"("Item Symbols"=w409) -> ()  [unwired: 2 in, 2 out]
          }
          frame Default {
          }
        }
      }
      event "Motor.Enable": Value Change {
        # "When the test mode otor enable helper is set, update that\ntree row item's value"
        n267 = event-data() -> ("NewVal"=w416:bool)  [unwired: 1 in]
        n268 = Unbundle("Motor") -> ("Value"=w415:dbl)  [unwired: 1 out]
        n269 = Select(t=w415, s=w416, f=0.0) -> (s? t:f=w413:dbl)
        n270 = call <vilib>:"NT Write Number.vi"("Numeric"=w413, "Name"=w412) -> ()  [unwired: 9 in, 1 out]
      }
      event "Test Slider": Value Change {
        # "When the test mode slider helper is set, update that\ntree row item's value"
        n271 = event-data() -> ("NewVal"=w419:dbl)  [unwired: 1 in]
        n272 = call <vilib>:"NT Write Number.vi"("Numeric"=w419, "Name"=w420) -> ()  [unwired: 9 in, 1 out]
      }
      event "On/Off": Value Change {
        # "When the test mode on/off helper value is set, update that\ntree row item's value"
        n273 = event-data() -> ("NewVal"=w424:bool)  [unwired: 1 in]
        n274 = Boolean To (0,1)(Boolean=w424) -> (0, 1=w423:i16)
        n275 = call <vilib>:"NT Write Number.vi"("Numeric"=w423, "Name"=w422) -> ()  [unwired: 9 in, 1 out]
      }
      event "Rev/Fwd": Value Change {
        # "When the test mode helper value for relays is set, update that\ntree row item's value"
        n276 = event-data() -> ("NewVal.Forward"=w432:bool, "NewVal.Reverse"=w431:bool)  [unwired: 1 in]
        n277 = Boolean To (0,1)(Boolean=w432) -> (0, 1=w428:i16)
        n278 = Boolean To (0,1)(Boolean=w431) -> (0, 1=w430:i16)
        n279 = Negate(x=w430) -> (-x=w429:i16)
        n280 = Add(x=w428, y=w429) -> (x+y=w427:i16)
        n281 = call <vilib>:"NT Write Number.vi"("Numeric"=w427, "Name"=w426) -> ()  [unwired: 9 in, 1 out]
      }
      event "Test Ring": Value Change {
        # "When a test mode helper value is selected from the ring,\nset the tree item's variable to the string value"
        n282 = event-data() -> ("NewVal"=w436:u16)  [unwired: 1 in]
        n283 = property on="Test Ring" class="Ring (strict)"() -> ("Strings []"=w437:string[])  [unwired: 2 in, 2 out]
        n284 = Index Array(array=w437, index=w436) -> (element=w435:string)
        n285 = call <vilib>:"NT Write String.vi"("String"=w435, "Name"=w434) -> ()  [unwired: 9 in, 1 out]
      }
      event "Rec Mode": Value Change {
        # "Update globals for recording mode and path to read log from.\nClear when logging and let NetworkTables set path for vision to\nuse."
        n286 = event-data() -> ("NewVal"=w448:enum32{"Stop", "Record", "Playback"})  [unwired: 1 in]
        n287 = global write "WPI_DashboardLogging Global.vi" "Logging Filename"(path "") -> ()
        n288 = global write "WPI_DashboardLogging Global.vi" "Recording"(w448) -> ()
        n289 = case shown="\"Playback\"" w448 {
          tunnel: w447 -> [_ w450 w459]
          tunnel: [_ _ w458] -> w445
          tunnel: [_ _ w457] -> _
          tunnel: w443 -> [_ _ w455]
          tunnel: cluster{i32, i32} {-250, 170} -> [_ _ w454]
          tunnel: [_ _ T20 {"Image Size"=TRUE, "Image Type"=TRUE, "Pixel Value"=TRUE, "ROI Information"=TRUE, "Zoom Factor"=FALSE} ("Image Information Shown:All Elements")] -> w441
          tunnel: [_ _ TRUE ("Zoom Factor")] -> w440
          tunnel: w439 -> [_ _ w451]
          frame Default {
          }
          frame "Stop", "Record" {
            # "Place Window too"
            n290 = invoke class="VI" method="FP.Close"(reference=w450) -> (reference out=w449:refnum<vi>)  [unwired: 2 in, 2 out]
            n291 = invoke class="VI" method="Abort VI"(reference=w449) -> ()  [unwired: 2 in, 3 out]
          }
          frame "Playback" {
            n292 = call "Open Playback Panel.vi"("Offset"=w454, "DB VI Ref"=w455, "Playback in"=w459) -> ("Playback out"=w456:refnum<vi>)  [unwired: 8 in]
            n293 = register-events(w456, w451) -> (reference out=w458:refnum<event-registration>, error out=w457:errorcluster)  [unwired: 2 in]
          }
        }
        n294 = property on="Camera Image" class="ImageControl"("Image Information Shown"=w441, "Image Information Visible"=w440) -> ()  [unwired: 2 in, 2 out]
        n295 = call <vilib>:"WPI_DashboardNT Log FieldName Cache.vi"("Operation"=enum16{"Lookup/Add", "Index", "Clear"}."Clear") -> ()  [unwired: 8 in, 3 out]
      }
      event Panel Close {
        w461 = enum32{"Stop", "Record", "Playback"}."Stop" ("Rec Mode")
        # "Playback window has been closed, abort"
        n296 = event-data() -> ()  [unwired: 1 in, 4 out]
        n297 = local write "Rec Mode"(w461) -> ()
        n298 = global write "WPI_DashboardLogging Global.vi" "Recording"(w461) -> ()
      }
      event Panel Close {
        # "Abort playback window and ourself"
        n299 = event-data() -> ()  [unwired: 1 in, 4 out]
        n300 = invoke class="VI" method="FP.Close"(reference=w465) -> (reference out=w464:refnum<vi>)  [unwired: 2 in, 2 out]
        n301 = invoke class="VI" method="Abort VI"(reference=w464) -> (error out=w463:errorcluster)  [unwired: 2 in, 2 out]
        n302 = invoke class="VI" method="Abort VI"(error in=w463) -> ()  [unwired: 2 in, 3 out]
      }
      event User Event {
        n303 = event-data() -> ("IDs"=w472:cluster{"RPC field ID":u16, "Unique ID":u16}, "String"=w471:string)  [unwired: 1 in]
        n304 = Bundle("IDs"=w472, "String"=w471) -> (w470:T8)  [unwired: 1 in]
        n305 = call <vilib>:"Retrieve RPC Response.vi"("RPC Response"=w470) -> ("Output"=w468:string[][])  [unwired: 10 in]
        n306 = Build Array (concatenate)(w466, w468) -> (w467:string[][])
        n307 = local write "Command Params"(w467) -> ()
        n308 = local write "Cmd Status"("" ("Cmd Status")) -> ()
      }
      event "Tree": Double Click {
        n309 = event-data() -> ("PlatMods"=w476:T23, "Tag"=w475:string)  [unwired: 1 in]
        n310 = Unbundle(w476) -> ("Shift"=w474:bool)  [unwired: 4 out]
        n311 = Not(x=w474) -> (.not. x?=w473:bool)
        n312 = call <vilib>:"NT Update Persistence.vi"("Persistence"=w473, "Name"=w475) -> ()  [unwired: 9 in, 1 out]
      }
    }
  }
  n313 = while {
    tunnel: w62 -> [w479]
    i -> [w482]
    stop <- FALSE stop-if-true
    n314 = Wait (ms)(milliseconds to wait=u32 100) -> ()  [unwired: 1 out]
    n315 = case shown="\"Playback\"" "Rec Mode" {
      tunnel: w482 -> [_ _ w497]
      tunnel: [u32 2829099 ("Base Color") u32 11141120 ("Target Color") w486] -> w478
      frame "Stop", Default {
        # "Reset the color, extra updates don't cost much"
      }
      frame "Record" {
      }
      frame "Playback" {
        # "Playback"
        n316 = Quotient & Remainder(x=w497, y=u32 50 ("milliseconds to wait")) -> (x-y*floor(x/y)=w493:u32)  [unwired: 1 out]
        n317 = Divide(x=w493, y=u32 50 ("milliseconds to wait")) -> (x/y=w490:dbl)
        n318 = Multiply(x=6.283185307179586, y=w490) -> (x*y=w495:dbl)
        n319 = Sine(x=w495) -> (sin(x)=w494:dbl)
        n320 = Absolute Value(x=w494) -> (abs(x)=w487:dbl)
        n321 = call "Interpolate RGB Color.vi"("Proportion"=w487, "Target Color"=u32 30976, "Base Color"=u32 2829099) -> ("Result Color"=w486:u32)  [unwired: 8 in]
      }
    }
    n322 = property class="Pane"(reference=w479, "PaneColor"=w478) -> ()  [unwired: 1 in, 2 out]
  }
  n323 = local write "Dashboard Tab"(T2."Drive" ("Dashboard Tab")) -> ()
  n324 = property on="On/Off" class="Bool (strict)"("Visible"=w31) -> ()  [unwired: 2 in, 2 out]
  n325 = property on="Motor" class="Clust (strict)"("Visible"=w31) -> ()  [unwired: 2 in, 2 out]
  n326 = property on="Progress" class="Clust (strict)"("Visible"=w31) -> ()  [unwired: 2 in, 2 out]
  n327 = property on="Test Ring" class="Ring (strict)"("Visible"=w31) -> ()  [unwired: 2 in, 2 out]
  n328 = property on="Rev/Fwd" class="Clust (strict)"("Visible"=w31) -> ()  [unwired: 2 in, 2 out]
  n329 = while {
    tunnel: u16 1741 ("timeout ms (25000)") -> [w499]
    stop <- FALSE stop-if-true
    n330 = TCP Create Listener(10:w499) -> (0:w498:errorcluster, 3:w500:refnum<k5>)  [unwired: 4 in, 1 out]
    n331 = case shown="No Error" w498 {
      selector: w498 -> [w502 _]
      tunnel: w500 -> [w503 _]
      frame No Error {
        n332 = while {
          tunnel: w503 -> [w506]
          tunnel: w502 -> [w505]
          stop <- FALSE stop-if-true
          n333 = TCP Wait On Listener(8:w505, 11:w506) -> (0:w507:errorcluster, 4:w508:refnum<k5>)  [unwired: 2 in, 3 out]
          n334 = local write "TCP"(w508) -> ()
          n335 = case shown="No Error" w507 {
            frame No Error {
            }
            frame Error {
              n336 = Wait (ms)(milliseconds to wait=u32 1000) -> ()  [unwired: 1 out]
            }
          }
        }
      }
      frame Error {
        n337 = Wait (ms)(milliseconds to wait=u32 1000) -> ()  [unwired: 1 out]
      }
    }
  }
  n338 = local write "Command Selection"(u16 0 ("milliseconds to wait")) -> ()
  n339 = local write "Command Params"(string[][] [] ("Command Params")) -> ()
  n340 = global write "WPI_DashboardLogging Global.vi" "Recording"(w56) -> ()
  n341 = local write "Rec Mode"(w56) -> ()
